vi "Open Spreadsheet subVI.vi"(8 "error in (no error)":errorcluster, 10 "FileStream":refnum<k24>, 11 "Excel XML in":refnum<class "Excel XML.lvclass">) -> (0 "error out":errorcluster, 3 "Excel XML out":refnum<class "Excel XML.lvclass">)   [LabVIEW 2013, in "Excel XML.lvclass"]
uses:
  Excel XML.lvclass
  C:/PhaeronGit/LVNPOI/Resources/NPOI 2.1.1 dotnet4/NPOI.OOXML.dll
  Resources/NPOI 2.1.1 dotnet4/NPOI.OOXML.dll
  Excel XML.lvclass/Excel XML.ctl
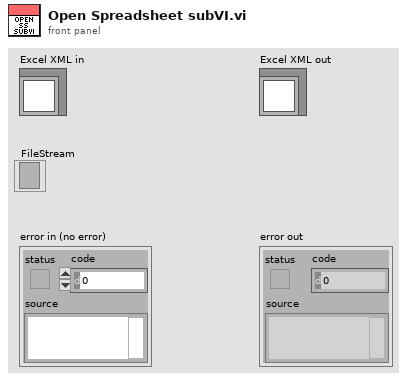
[diagram p1: front panel]
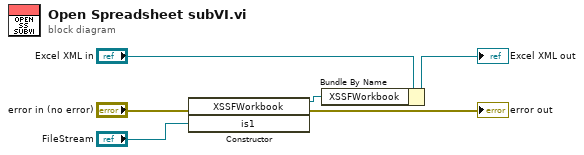
[diagram p0: block diagram]
diagram:
  n1 = constructor class="XSSFWorkbook"(error in="error in (no error)", "is1"="FileStream") -> (reference out=w4:refnum<k24>, error out=→"error out":errorcluster)  [unwired: 2 in, 2 out]
  n2 = Bundle By Name(cluster="Excel XML in", "XSSFWorkbook"=w4) -> (→"Excel XML out":refnum<class "Excel XML.lvclass">)
